vi "Bridgewire Measurement.vi"(0 "Valhalla Resource Name":refnum<visa-resource-name>="COM12", 5 "Switch Resource Name":refnum<visa-resource-name>="COM12", 9 "upper resistance limit":dbl, 11 "error in (no error)":errorcluster, 12 "lower resistance limit":dbl) -> (1 "Stop Status":bool, 2 "BW1 Resistance Result":u16, 3 "BW1 In Tolerance?":bool, 4 "Test Status":string, 6 "BW 1 Resistance":string, 10 "BW 2 Resistance":string, 13 "BW2 Resistance Result":u16, 14 "BW2 In Tolerance?":bool, 15 "error out":errorcluster)   [LabVIEW 2018]
uses:
  Custom Controls/Bridgewire Resistance Test State.ctl
  Door Status Global Variable.vi
  Agilent 34970/Agilent 34970.lvlib
panel:
  in  "BW Resistance Test State":T1=enum."BW Resistance 1"
  out "Current Range":string
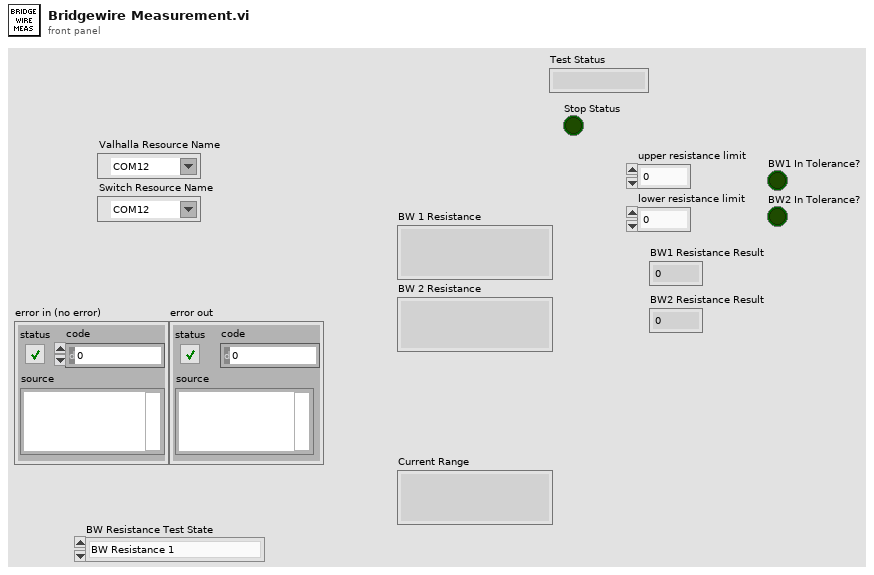
[diagram p1: front panel]
types:
  T1 = typedef "Bridgewire Resistance Test State.ctl" = enum16{"Initialize", "Switch for BW 1", "BW Resistance 1", "Switch for BW 2", "BW Resistance 2", "User Stop", "Stop"}
  T2 = enum16{"None", "XON / XOFF", "RTS / CTS", "DTR / DSR"}
  T3 = enum16{"1200", "2400", "4800", "9600", "19200", "38400", "57600", "115200"}
  T4 = cluster{"Timeout Value (10000)":u32, "Baud Rate (57600)":enum16{"1200", "2400", "4800", "9600", "19200", "38400", "57600", "115200"}, "Flow Control (1:XON/XOFF)":enum16{"None", "XON / XOFF", "RTS / CTS", "DTR / DSR"}}
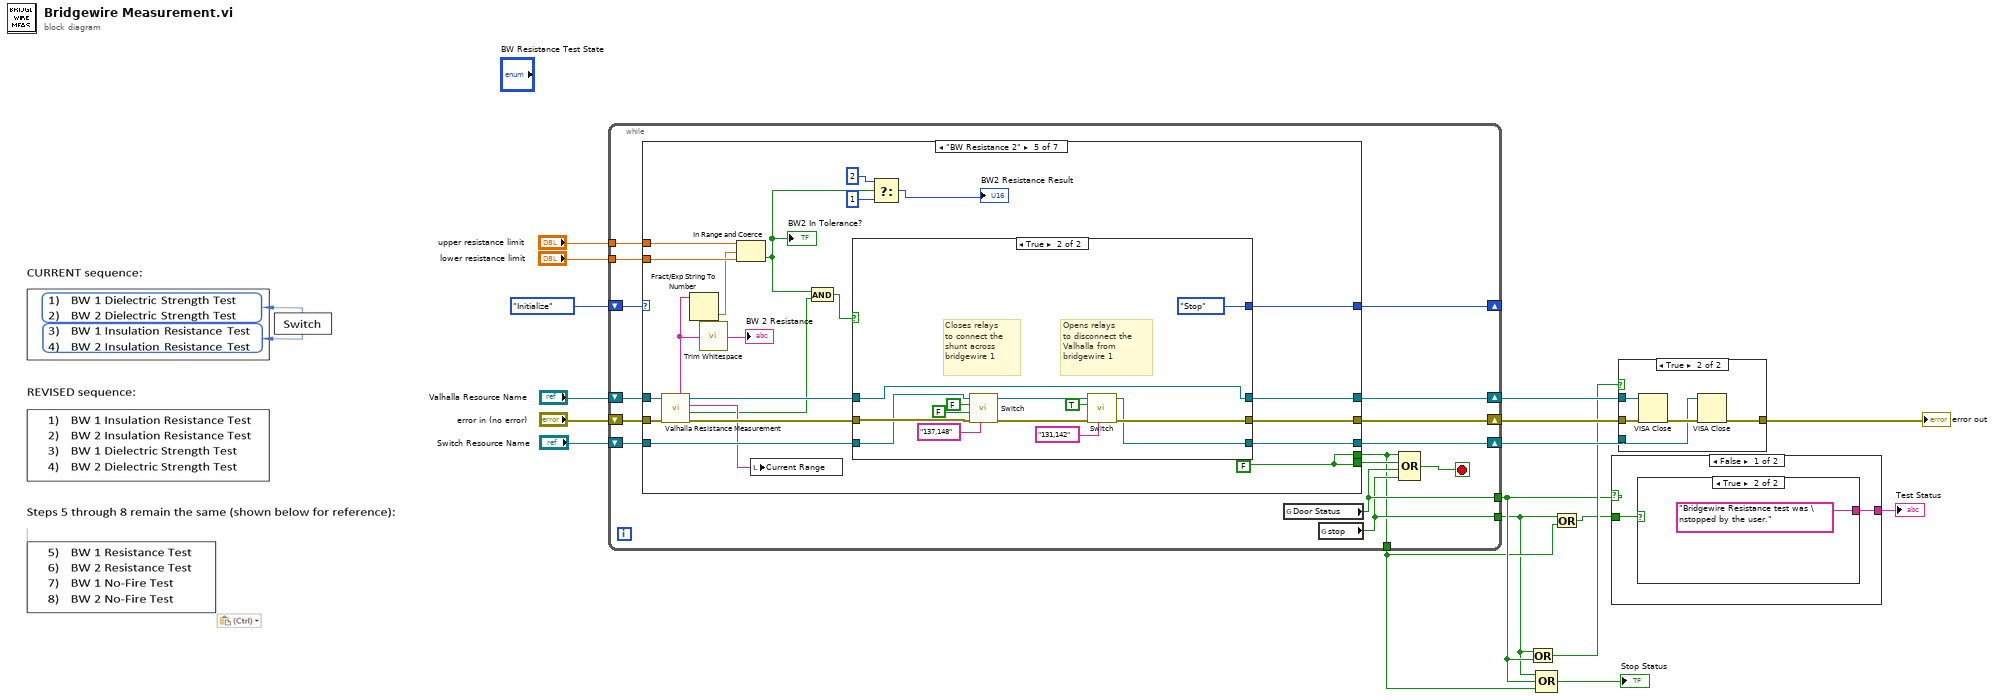
[diagram p0: block diagram]
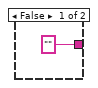
[diagram p3: hidden frame]
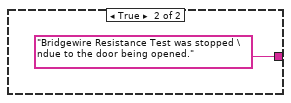
[diagram p4: hidden frame]
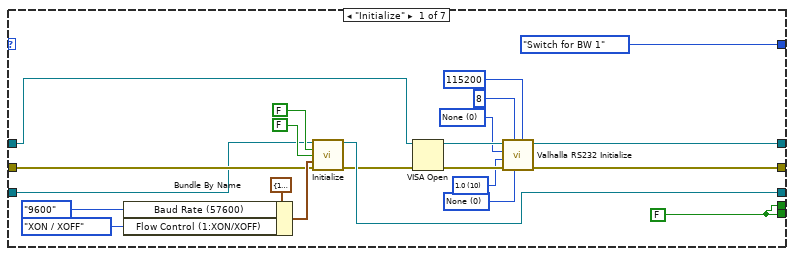
[diagram p5: hidden frame]
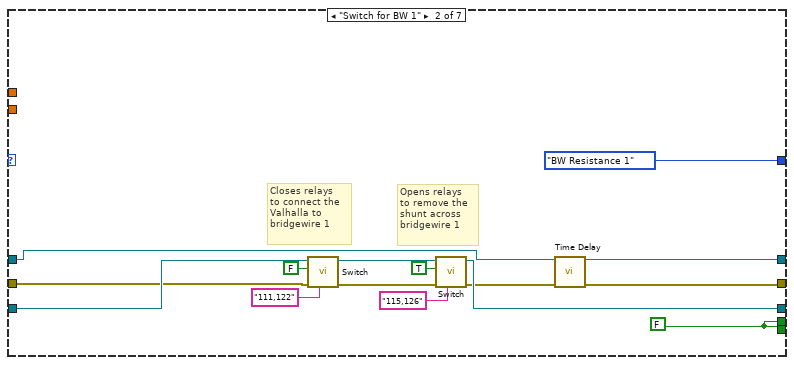
[diagram p6: hidden frame]
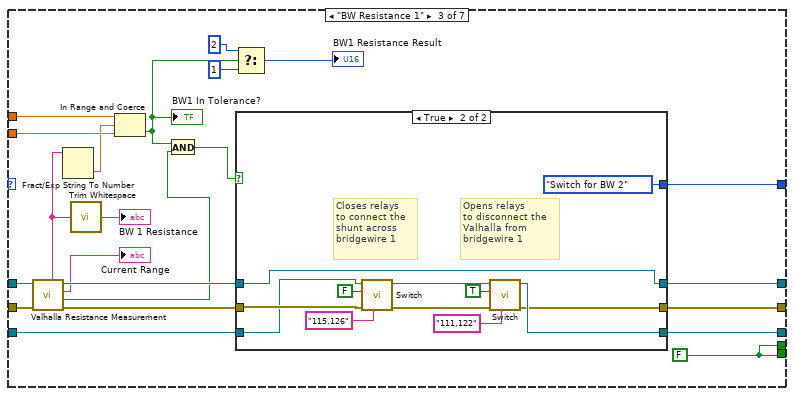
[diagram p7: hidden frame]
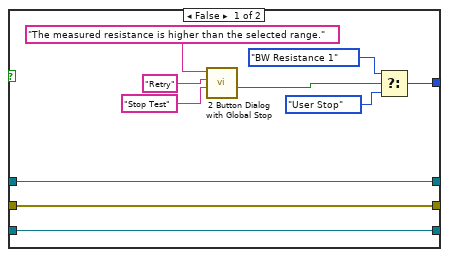
[diagram p8: hidden frame]
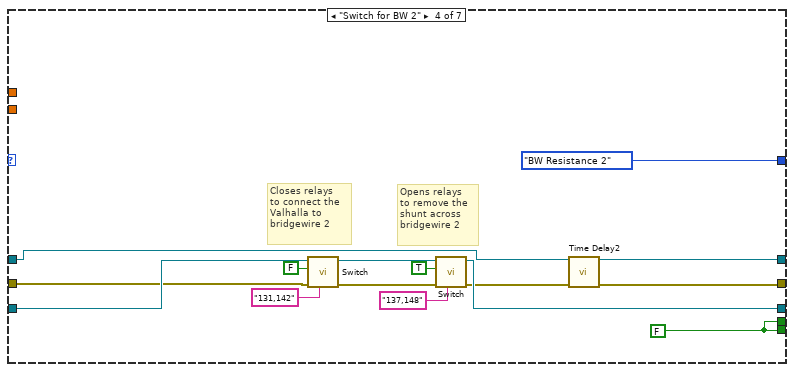
[diagram p9: hidden frame]
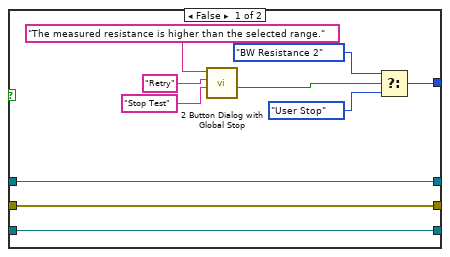
[diagram p10: hidden frame]
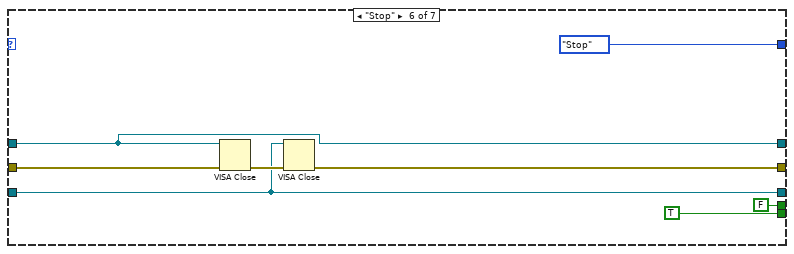
[diagram p11: hidden frame]
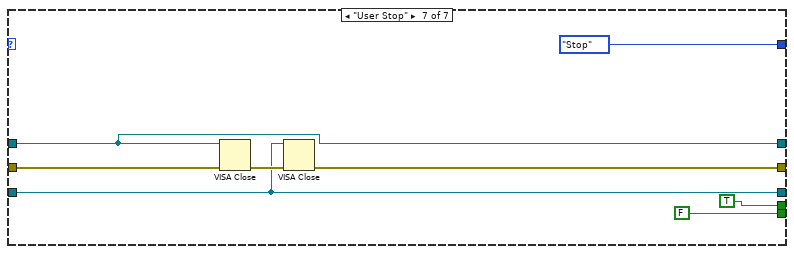
[diagram p12: hidden frame]
diagram:
  n1 = while {
    shift-right: [w31] -> w8
    shift-left: "error in (no error)" -> [w32]
    shift-right: [w29] -> w10
    shift-left: "Valhalla Resource Name" -> [w30]
    shift-right: [w27] -> _
    shift-left: Bridgewire_Resistance_Test_State."Initialize" ("BW Resistance Test State") -> [w23]
    shift-right: [w26] -> w9
    shift-left: "Switch Resource Name" -> [w28]
    tunnel: "upper resistance limit" -> [w25]
    tunnel: "lower resistance limit" -> [w24]
    tunnel: [w21] -> w5
    tunnel: [w19] -> w2
    tunnel: [w18] -> w3
    stop <- w20 stop-if-true
    n2 = case shown="\"BW Resistance 2\"" w23 {
      tunnel: [Bridgewire_Resistance_Test_State."Switch for BW 1" ("BW Resistance Test State") Bridgewire_Resistance_Test_State."BW Resistance 1" ("BW Resistance Test State") w90 Bridgewire_Resistance_Test_State."BW Resistance 2" ("BW Resistance Test State") w148 Bridgewire_Resistance_Test_State."Stop" ("BW Resistance Test State") Bridgewire_Resistance_Test_State."Stop" ("BW Resistance Test State")] -> w27
      tunnel: w32 -> [w40 w61 w89 w119 w147 w177 w186]
      tunnel: [w47 w57 w84 w115 w142 w176 w185] -> w31
      tunnel: w30 -> [w39 w59 w88 w117 w146 w174 w183]
      tunnel: [w46 w59 w85 w117 w143 w174 w183] -> w29
      tunnel: w28 -> [w35 w67 w83 w125 w141 w175 w184]
      tunnel: [w38 w60 w82 w118 w140 w175 w184] -> w26
      tunnel: [w33 w55 w73 w113 w133 TRUE FALSE] -> w22
      tunnel: w25 -> [_ _ w79 _ w138 _ _]
      tunnel: w24 -> [_ _ w80 _ w137 _ _]
      tunnel: [w33 w55 w73 w113 w133 FALSE TRUE] -> w18
      frame "Initialize" {
        w33 = FALSE
        w50 = u16 10 items=["1.0"=10, "1.5"=15, "2.0"=20] ("Stop Bits")
        w49 = u16 0 items=["None", "Odd", "Even", "Mark", "Space"] ("Parity")
        w52 = u16 0 items=["None", "XON/XOFF", "RTS/CTS", "XON/XOFF & RTS/CTS", "DTR/DSR", "XON/XOFF & DTR/DSR"] ("Flow Control")
        n3 = Bundle By Name(cluster=T4 {"Timeout Value (10000)"=10000, "Baud Rate (57600)"=enum."9600", "Flow Control (1:XON/XOFF)"=enum."XON / XOFF"} ("Serial Port Configuration"), "Baud Rate (57600)"=T3."9600", "Flow Control (1:XON/XOFF)"=T2."XON / XOFF") -> (w44:T4)
        n4 = call "Initialize.vi"("VISA Resource Name"=w35, "ID Query (T: Check)"=FALSE, "Reset (T: Reset)"=FALSE, "Serial Port Configuration"=w44, "error in (no error)"=w40) -> ("VISA Resource Name Out"=w38:refnum<visa-resource-name>, "error out"=w37:errorcluster)  [unwired: 9 in]
        n5 = VISA Open(error in (no error)=w37, VISA resource name=w39) -> (VISA resource name=w53:refnum<visa-resource-name>, error out=w54:errorcluster)  [unwired: 3 in]
        n6 = call "Valhalla RS232 Initialize.vi"("Baud Rate"=u32 115200, "Flow Control"=w52, "Data Bits"=u16 8, "error in (no error)"=w54, "Stop Bits"=w50, "Parity"=w49, "VISA Refnum in"=w53) -> ("error out"=w47:errorcluster, "VISA Refnum out"=w46:refnum<visa-resource-name>)  [unwired: 3 in]
      }
      frame "Switch for BW 1" {
        w55 = FALSE
        # "Opens relays\nto remove the \nshunt across \nbridgewire 1"
        # "Closes relays\nto connect the \nValhalla to \nbridgewire 1"
        n7 = call "Switch.vi"("Channel List(empty)"="111,122", "error in (no error)"=w61, "Open/Close (F:Close)"=FALSE, "VISA Resource Name"=w67) -> ("error out"=w62:errorcluster, "VISA Resource Name Out"=w64:refnum<visa-resource-name>)  [unwired: 5 in, 1 out]
        n8 = call "Switch.vi"("Channel List(empty)"="115,126", "error in (no error)"=w62, "Open/Close (F:Close)"=TRUE, "VISA Resource Name"=w64) -> ("error out"=w58:errorcluster, "VISA Resource Name Out"=w60:refnum<visa-resource-name>)  [unwired: 5 in, 1 out]
        n9 = call "Time Delay"("error in (no error)"=w58) -> ("error out"=w57:errorcluster)  [unwired: 10 in]
      }
      frame "BW Resistance 1" {
        w73 = FALSE
        n10 = call "Valhalla Resistance Measurement.vi"("error in (no error)"=w89, "VISA Refnum in"=w88) -> ("error out"=w86:errorcluster, "In Range?"=w75:bool, "Current Range"=→"Current Range":string, "VISA Refnum out"=w87:refnum<visa-resource-name>, "Resistance"=w77:string)  [unwired: 5 in]
        n11 = Fract/Exp String To Number(string=w77) -> (number=w78:dbl)  [unwired: 3 in, 1 out]
        n12 = call <vilib>:"Trim Whitespace.vi"("string"=w77) -> ("trimmed string"=→"BW 1 Resistance":string)  [unwired: 1 in]
        n13 = In Range and Coerce(upper limit=w79, x=w78, lower limit=w80) -> (In Range?=w72:bool)  [unwired: 1 out]
        "BW1 In Tolerance?" <- w72
        n14 = And(x=w72, y=w75) -> (x .and. y?=w74:bool)
        n15 = Select(t=u16 2 ("BW1 Resistance Result"), s=w72, f=u16 1) -> (s? t:f=→"BW1 Resistance Result":u16)
        n16 = case shown="True" w74 {
          tunnel: [w98 Bridgewire_Resistance_Test_State."Switch for BW 2" ("BW Resistance Test State")] -> w90
          tunnel: w87 -> [w97 w103]
          tunnel: w86 -> [w96 w106]
          tunnel: [w97 w103] -> w85
          tunnel: [w96 w102] -> w84
          tunnel: w83 -> [w95 w105]
          tunnel: [w95 w104] -> w82
          frame False {
            n17 = call "2 Button Dialog with Global Stop.vi"("F Button Name (\"CANCEL\")"="Stop Test" ("F button name (\"Cancel\")"), "T Button Name (\"OK\")"="Retry" ("T button name (\"OK\")"), "Dialog Message"="The measured resistance is higher than the selected range." ("message")) -> ("Global Stop?"=w99:bool)  [unwired: 6 in, 2 out]
            n18 = Select(t=Bridgewire_Resistance_Test_State."BW Resistance 1" ("BW Resistance Test State"), s=w99, f=Bridgewire_Resistance_Test_State."User Stop" ("BW Resistance Test State")) -> (s? t:f=w98:T1)
          }
          frame True {
            # "Closes relays\nto connect the \nshunt across \nbridgewire 1"
            # "Opens relays\nto disconnect the \nValhalla from \nbridgewire 1"
            n19 = call "Switch.vi"("Channel List(empty)"="115,126", "error in (no error)"=w106, "Open/Close (F:Close)"=FALSE, "VISA Resource Name"=w105) -> ("error out"=w112:errorcluster, "VISA Resource Name Out"=w111:refnum<visa-resource-name>)  [unwired: 5 in, 1 out]
            n20 = call "Switch.vi"("Channel List(empty)"="111,122", "error in (no error)"=w112, "Open/Close (F:Close)"=TRUE, "VISA Resource Name"=w111) -> ("error out"=w102:errorcluster, "VISA Resource Name Out"=w104:refnum<visa-resource-name>)  [unwired: 5 in, 1 out]
          }
        }
      }
      frame "Switch for BW 2" {
        w113 = FALSE
        # "Opens relays\nto remove the \nshunt across \nbridgewire 2"
        # "Closes relays\nto connect the \nValhalla to \nbridgewire 2"
        n21 = call "Switch.vi"("Channel List(empty)"="131,142", "error in (no error)"=w119, "Open/Close (F:Close)"=FALSE, "VISA Resource Name"=w125) -> ("error out"=w120:errorcluster, "VISA Resource Name Out"=w122:refnum<visa-resource-name>)  [unwired: 5 in, 1 out]
        n22 = call "Switch.vi"("Channel List(empty)"="137,148", "error in (no error)"=w120, "Open/Close (F:Close)"=TRUE, "VISA Resource Name"=w122) -> ("error out"=w116:errorcluster, "VISA Resource Name Out"=w118:refnum<visa-resource-name>)  [unwired: 5 in, 1 out]
        n23 = call "Time Delay2"("error in (no error)"=w116) -> ("error out"=w115:errorcluster)  [unwired: 10 in]
      }
      frame "BW Resistance 2" {
        w133 = FALSE
        n24 = call "Valhalla Resistance Measurement.vi"("error in (no error)"=w147, "VISA Refnum in"=w146) -> ("error out"=w144:errorcluster, "In Range?"=w132:bool, "Current Range"=w139:string, "VISA Refnum out"=w145:refnum<visa-resource-name>, "Resistance"=w135:string)  [unwired: 5 in]
        n25 = Fract/Exp String To Number(string=w135) -> (number=w136:dbl)  [unwired: 3 in, 1 out]
        n26 = call <vilib>:"Trim Whitespace.vi"("string"=w135) -> ("trimmed string"=→"BW 2 Resistance":string)  [unwired: 1 in]
        n27 = In Range and Coerce(upper limit=w138, x=w136, lower limit=w137) -> (In Range?=w128:bool)  [unwired: 1 out]
        "BW2 In Tolerance?" <- w128
        n28 = local write "Current Range"(w139) -> ()
        n29 = And(x=w128, y=w132) -> (x .and. y?=w131:bool)
        n30 = case shown="True" w131 {
          tunnel: [w156 Bridgewire_Resistance_Test_State."Stop" ("BW Resistance Test State")] -> w148
          tunnel: w145 -> [w155 w161]
          tunnel: w144 -> [w154 w165]
          tunnel: [w155 w161] -> w143
          tunnel: [w154 w164] -> w142
          tunnel: w141 -> [w153 w163]
          tunnel: [w153 w162] -> w140
          frame False {
            n31 = call "2 Button Dialog with Global Stop.vi"("F Button Name (\"CANCEL\")"="Stop Test" ("F button name (\"Cancel\")"), "T Button Name (\"OK\")"="Retry" ("T button name (\"OK\")"), "Dialog Message"="The measured resistance is higher than the selected range." ("message")) -> ("Global Stop?"=w157:bool)  [unwired: 6 in, 2 out]
            n32 = Select(t=Bridgewire_Resistance_Test_State."BW Resistance 2" ("BW Resistance Test State"), s=w157, f=Bridgewire_Resistance_Test_State."User Stop" ("BW Resistance Test State")) -> (s? t:f=w156:T1)
          }
          frame True {
            # "Closes relays\nto connect the \nshunt across \nbridgewire 1"
            # "Opens relays\nto disconnect the \nValhalla from \nbridgewire 1"
            n33 = call "Switch.vi"("Channel List(empty)"="137,148", "error in (no error)"=w165, "Close Exclusive (F:Normal)"=FALSE, "Open/Close (F:Close)"=FALSE, "VISA Resource Name"=w163) -> ("error out"=w171:errorcluster, "VISA Resource Name Out"=w170:refnum<visa-resource-name>)  [unwired: 4 in, 1 out]
            n34 = call "Switch.vi"("Channel List(empty)"="131,142", "error in (no error)"=w171, "Open/Close (F:Close)"=TRUE, "VISA Resource Name"=w170) -> ("error out"=w164:errorcluster, "VISA Resource Name Out"=w162:refnum<visa-resource-name>)  [unwired: 5 in, 1 out]
          }
        }
        n35 = Select(t=u16 2 ("BW1 Resistance Result"), s=w128, f=u16 1) -> (s? t:f=→"BW2 Resistance Result":u16)
      }
      frame "Stop" {
        n36 = VISA Close(VISA resource name=w174, error in (no error)=w177) -> (error out=w178:errorcluster)
        n37 = VISA Close(VISA resource name=w175, error in (no error)=w178) -> (error out=w176:errorcluster)
      }
      frame "User Stop" {
        n38 = VISA Close(VISA resource name=w183, error in (no error)=w186) -> (error out=w187:errorcluster)
        n39 = VISA Close(VISA resource name=w184, error in (no error)=w187) -> (error out=w185:errorcluster)
      }
    }
    n40 = global read "Door Status Global Variable.vi" "Door Status"() -> (w21:bool)
    n41 = global read "Door Status Global Variable.vi" "stop"() -> (w19:bool)
    n42 = Compound Arithmetic op=OR(w18, w22, w21, w19) -> (w20:bool)
  }
  n43 = Or(x=w2, y=w5) -> (x .or. y?=w6:bool)
  n44 = Compound Arithmetic op=OR(w2, w5, w3) -> (→"Stop Status":bool)
  n45 = Or(x=w2, y=w3) -> (x .or. y?=w1:bool)
  n46 = case shown="False" w5 {
    tunnel: [w188 "Bridgewire Resistance Test was stopped \ndue to the door being opened." ("Test Status")] -> w11
    tunnel: w1 -> [w189 _]
    frame False {
      n47 = case shown="True" w189 {
        tunnel: ["" ("Test Status") "Bridgewire Resistance test was \nstopped by the user." ("Test Status")] -> w188
        frame False {
        }
        frame True {
        }
      }
    }
    frame True {
    }
  }
  "Test Status" <- w11
  n48 = case shown="True" w6 {
    tunnel: w10 -> [_ w197]
    tunnel: w9 -> [_ w196]
    tunnel: w8 -> [w193 w195]
    tunnel: [w193 w194] -> w7
    frame False {
    }
    frame True {
      n49 = VISA Close(VISA resource name=w197, error in (no error)=w195) -> (error out=w198:errorcluster)
      n50 = VISA Close(VISA resource name=w196, error in (no error)=w198) -> (error out=w194:errorcluster)
    }
  }
  "error out" <- w7
